vi "Get or Create Server Reference.vi"(8 "error in (no error)":errorcluster) -> (0 "error out":errorcluster, 3 "Server Out":refnum<class "JSONRPC Server.lvclass">)   [LabVIEW 2020, in "JSON-RPC Lib.lvlib" / "JSONRPC Server.lvclass"]
doc: "If no other RPC Servers are running in this application instance, this initializes the server. If there are other server references active, this duplicates the existing server reference."
uses:
  JSONRPC Server.lvclass
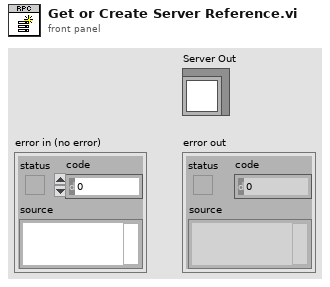
[diagram p1: front panel]
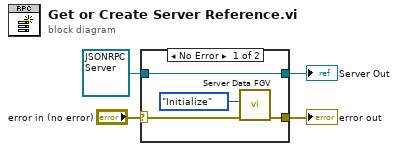
[diagram p0: block diagram]
diagram:
  n1 = case shown="No Error" "error in (no error)" {
    selector: "error in (no error)" -> [w8 w10]
    tunnel: [w7 w10] -> w3
    tunnel: [w6 w9] -> w2
    tunnel: refnum<class "JSONRPC Server.lvclass"> refnum ("Server.lvclass") -> [w6 w9]
    frame No Error {
      n2 = call "Server Data FGV.vi"("error in (no error)"=w8, "Action"=enum16{"Initialize", "Check", "Close"}."Initialize") -> ("error out"=w7:errorcluster)  [unwired: 6 in, 3 out]
    }
    frame Error {
    }
  }
  "error out" <- w3
  "Server Out" <- w2
